vi "GlobalPyConsole.vi"() -> ()   [LabVIEW 2019, in "Global.lvlib"]
uses:
  Global.lvlib
panel:
  out "Python Console":string
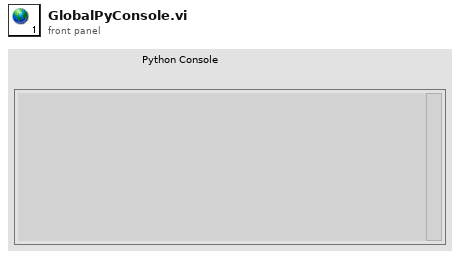
[diagram p1: front panel]
diagram:
